vi "Trapezoidal Profile Lookup Setpoints.vi"(10 "Total Distance":sgl, 11 "Current Time":u32) -> (2 "Acceleration":sgl, 3 "Velocity":sgl, 5 "Profile Completed?":bool)   [LabVIEW 2015]
uses:
  Trapezoidal Motion State.ctl
panel:
  out "Stage 2 Time":sgl
  out "Stage 3 Time":sgl
  out "Stage 1 Time":sgl
  out "Max Reachable Velocity":sgl
  out "Cruise Velocity":sgl
  out "Total Time":sgl
  in  "Max Velocity":sgl=13.5
  in  "Acceleration":sgl=6.0
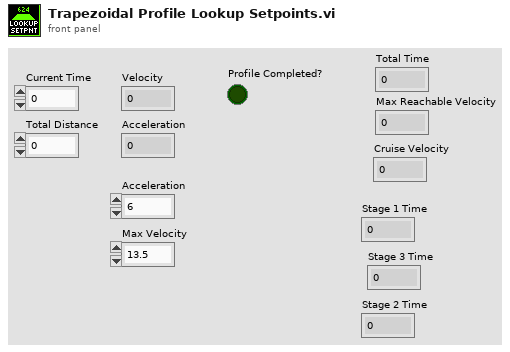
[diagram p1: front panel]
types:
  T1 = typedef "Trapezoidal Motion State.ctl" = enum16{"Accelerate", "Cruise", "Decelerate", "Finish"}
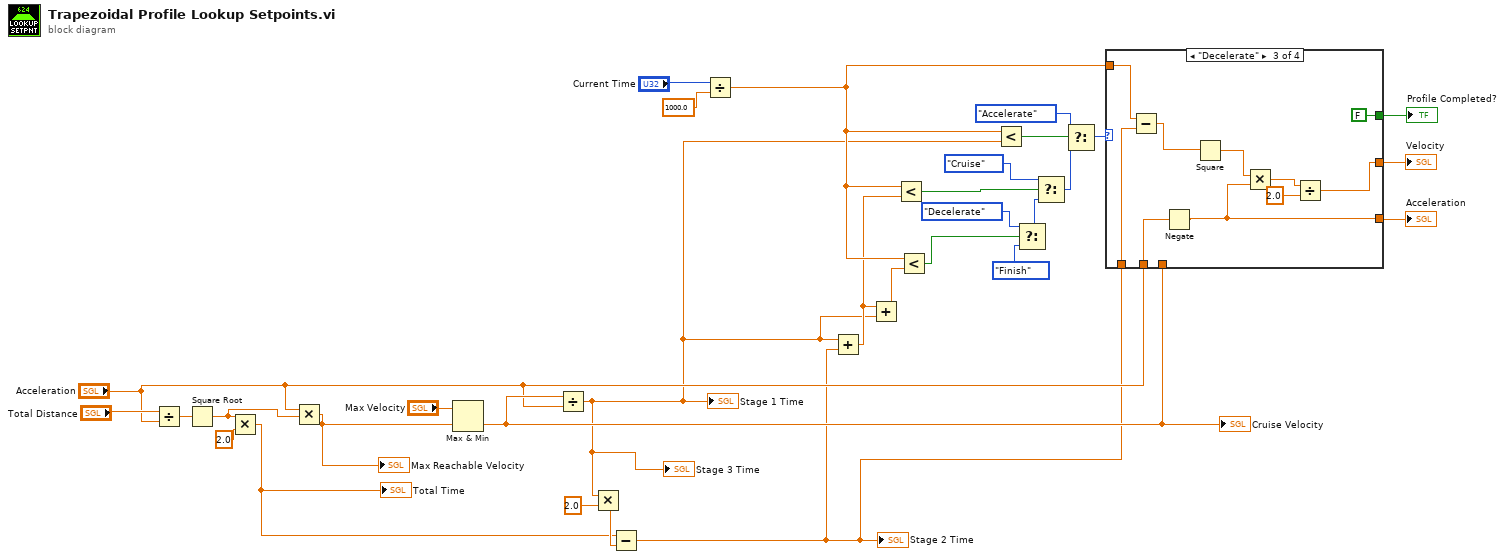
[diagram p0: block diagram]
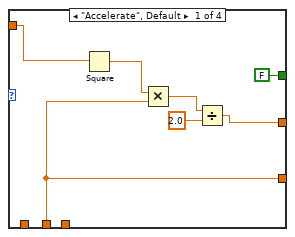
[diagram p2: hidden frame]
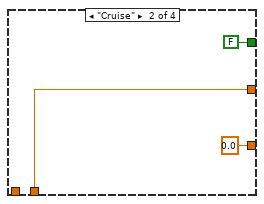
[diagram p3: hidden frame]
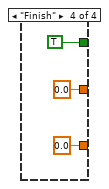
[diagram p4: hidden frame]
diagram:
  n1 = Divide(x="Total Distance", y="Acceleration") -> (x/y=w18:sgl)
  n2 = Square Root(x=w18) -> (sqrt(x)=w16:sgl)
  n3 = Multiply(x=w16, y=sgl 2.0) -> (x*y=w7:sgl)
  "Total Time" <- w7
  n4 = Multiply(x="Acceleration", y=w16) -> (x*y=w15:sgl)
  "Max Reachable Velocity" <- w15
  n5 = Max & Min(x="Max Velocity", y=w15) -> (min(x,y)=w13:sgl)  [unwired: 1 out]
  "Cruise Velocity" <- w13
  n6 = Divide(x=w13, y="Acceleration") -> (x/y=w3:sgl)
  "Stage 1 Time" <- w3
  "Stage 3 Time" <- w3
  n7 = Multiply(x=w3, y=sgl 2.0) -> (x*y=w10:sgl)
  n8 = Subtract(x=w7, y=w10) -> (x-y=w1:sgl)
  "Stage 2 Time" <- w1
  n9 = Divide(x="Current Time", y=sgl 1000.0) -> (x/y=w5:sgl)
  n10 = Add(x=w3, y=w1) -> (x+y=w4:sgl)
  n11 = Add(x=w4, y=w3) -> (x+y=w2:sgl)
  n12 = Less?(x=w5, y=w4) -> (x < y?=w29:bool)
  n13 = Less?(x=w5, y=w2) -> (x < y?=w26:bool)
  n14 = Less?(x=w5, y=w3) -> (x < y?=w31:bool)
  n15 = Select(t=Trapezoidal_Motion_State."Decelerate" ("Enum"), s=w26, f=Trapezoidal_Motion_State."Finish" ("Enum")) -> (s? t:f=w24:T1)
  n16 = Select(t=Trapezoidal_Motion_State."Cruise" ("Enum"), s=w29, f=w24) -> (s? t:f=w28:T1)
  n17 = Select(t=Trapezoidal_Motion_State."Accelerate" ("Enum"), s=w31, f=w28) -> (s? t:f=w23:T1)
  n18 = case shown="\"Decelerate\"" w23 {
    tunnel: [FALSE FALSE FALSE TRUE] -> w22
    tunnel: [w35 w39 w47 sgl 0.0 ("Cruise Velocity")] -> w21
    tunnel: [w33 sgl 0.0 ("Acceleration 3") w44 sgl 0.0 ("Acceleration 3")] -> w20
    tunnel: w5 -> [w32 _ w51 _]
    tunnel: w13 -> [_ w39 _ _]
    tunnel: "Acceleration" -> [w33 _ w45 _]
    tunnel: w1 -> [_ _ w42 _]
    frame "Accelerate", Default {
      n19 = Square(x=w32) -> (x^2=w38:sgl)
      n20 = Multiply(x=w38, y=w33) -> (x*y=w37:sgl)
      n21 = Divide(x=w37, y=sgl 2.0) -> (x/y=w35:sgl)
    }
    frame "Cruise" {
    }
    frame "Decelerate" {
      n22 = Subtract(x=w51, y=w42) -> (x-y=w43:sgl)
      n23 = Negate(x=w45) -> (-x=w44:sgl)
      n24 = Square(x=w43) -> (x^2=w50:sgl)
      n25 = Multiply(x=w50, y=w44) -> (x*y=w49:sgl)
      n26 = Divide(x=w49, y=sgl 2.0) -> (x/y=w47:sgl)
    }
    frame "Finish" {
    }
  }
  "Velocity" <- w21
  "Acceleration" <- w20
  "Profile Completed?" <- w22
